vi "AnalysatorAuswahl Ring befuellen.vi"(8 "error in (no error)":errorcluster caption="Fehler (Eingang, kein Fehler)", 10 "Strings und Werte []":T1, 11 "Ring (Eingang)":refnum<vi>) -> (0 "error out":errorcluster caption="Fehler (Ausgang)")   [LabVIEW 2020, in "System Einstellungen V2.lvlib"]
uses:
  System Einstellungen V2.lvlib
  <vilib>/Utility/miscctls.llb/LVComboBoxStrsAndValuesArrayTypeDef.ctl
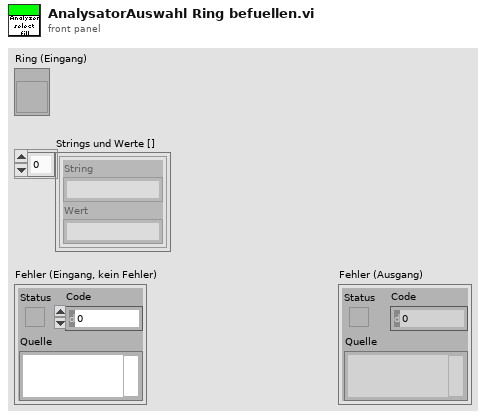
[diagram p1: front panel]
types:
  T1 = typedef "LVComboBoxStrsAndValuesArrayTypeDef.ctl" = cluster{"String":string, "Value":string}[]
  T2 = cluster{"Value":string, "Fließkommazahl (Single)":i16}[]
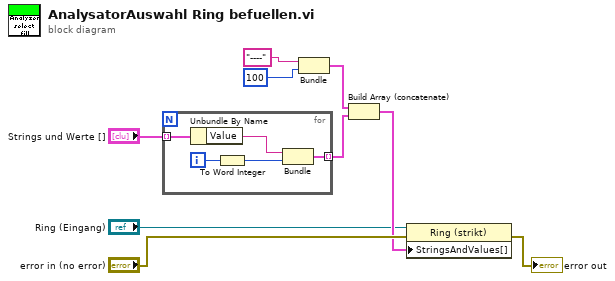
[diagram p0: block diagram]
diagram:
  n1 = for {
    tunnel: "Strings und Werte []" -> [w14] mode=indexing
    tunnel: [w12] -> w5 mode=indexing
    i -> [w13]
    n2 = Unbundle By Name(w14) -> ("Value"=w11:string)
    n3 = To Word Integer(number=w13) -> (16bit integer=w10:i16)
    n4 = Bundle("Value"=w11, w10) -> (w12:cluster{"Value":string, i16})  [unwired: 1 in]
  }
  n5 = Bundle("----", "Fließkommazahl (Single)"=i16 100) -> (w6:cluster{string, "Fließkommazahl (Single)":i16})  [unwired: 1 in]
  n6 = Build Array (concatenate)(w6, w5) -> (w4:T2)
  n7 = property class="Ring (strikt)"(reference="Ring (Eingang)", error in="error in (no error)", "StringsAndValues[]"=w4) -> (error out=→"error out":errorcluster)  [unwired: 1 out]
